vi "Pick Red.vi"(1 "Intensity (%)":dbl(slide) scale=0.0..100.0) -> (0 "Red Hue":u32(colorbox))   [LabVIEW 2016]
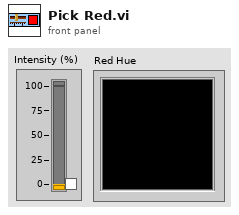
[diagram p1: front panel]
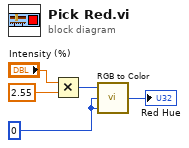
[diagram p0: block diagram]
diagram:
  w1 = u8 0 ("R")
  n1 = Multiply(x="Intensity (%)", y=2.55) -> (x*y=w2:u8)
  n2 = call <vilib>:"RGB to Color.vi"("B"=w1, "G"=w1, "R"=w2) -> ("Color"=→"Red Hue":u32)
